vi "General Polynomial Fit (LS).vi"(0 "Y":dbl[](array[numeric]), 1 "polynomial order":i32=2, 2 "Coefficient Constraint":cluster{"order":i32, "coefficient":dbl}[](array[cluster]), 5 "X":dbl[](array[numeric]), 7 "Weight":dbl[](array[numeric]), 13 "algorithm":T1 items=["SVD", "Givens", "Givens2", "Householder", "LU Decomposition", "Cholesky", "SVD for Rank Deficient H"]) -> (4 "Best Polynomial Fit":dbl[](array[numeric]), 6 "Polynomial Coefficients":dbl[](array[numeric]), 14 "mse":dbl, 15 "error":i32)   [LabVIEW 2010, in "NI_AALPro.lvlib"]
uses:
  NI_AALPro.lvlib
  General Linear Fit Algorithm.ctl
  lvanlys.dll
panel:
  # "LS General Polynomial Fit"
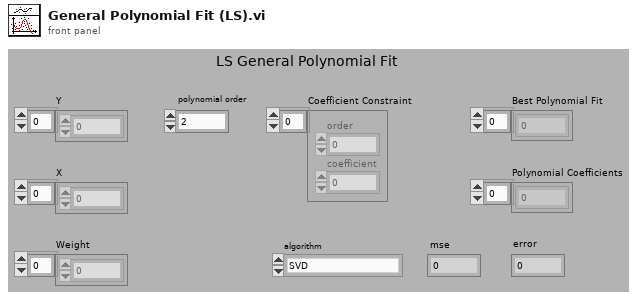
[diagram p1: front panel]
types:
  T1 = typedef "NI_AALPro.lvlib/General Linear Fit Algorithm.ctl" = u16
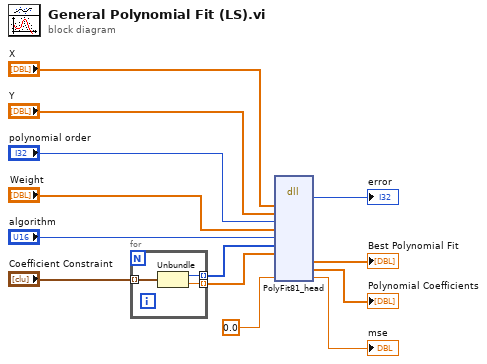
[diagram p0: block diagram]
diagram:
  n1 = for {
    tunnel: "Coefficient Constraint" -> [w16] mode=indexing
    tunnel: [w15] -> w3 mode=indexing
    tunnel: [w14] -> w4 mode=indexing
    n2 = Unbundle(w16) -> ("order"=w15:i32, "coefficient"=w14:dbl)
  }
  n3 = dll-call lib="C:/Program Files/National Instruments/LabVIEW 2010/resource/lvanlys.*" fn="PolyFit81_head"("xH"="X", "yH"="Y", "Order"="polynomial order", "weightH"="Weight", "algorithm"="algorithm", "specOrderH"=w3, "specCoefH"=w4, "mse"=0.0) -> ("return type"=→"error":i32, "BestFitH"=→"Best Polynomial Fit":dbl[], "CoefH"=→"Polynomial Coefficients":dbl[], "mse"=→"mse":dbl)  [unwired: 10 in, 4 out]
